vi "Chessy_Drive_Main.vi"(0 "Speed_Main":dbl, 1 "Turning_Main":dbl, 5 "Speed_Limit":dbl, 7 "Turning_Limit":dbl, 12 "Quick_Turn":bool) -> (3 "Left_Motor":dbl format="%.2f", 14 "Right_Motor":dbl format="%.2f")   [LabVIEW 2013]
panel:
  in  "Turning Scale":dbl=1.5
  in  "Turning Y":dbl[](array[numeric])=[-1.0, -0.5, -0.21, 0.0, 0.0, 0.0, 0.21, 0.5, 1.0]
  in  "Turning X":dbl[](array[numeric])=[-1.0, -0.75, -0.155, -0.15, 0.0, 0.15, 0.155, 0.75, 1.0]
  in  "Speed Y":dbl[](array[numeric])=[-1.0, -0.5, -0.21, 0.0, 0.0, 0.0, 0.21, 0.5, 1.0]
  in  "Speed X":dbl[](array[numeric])=[-1.0, -0.75, -0.155, -0.15, 0.0, 0.15, 0.155, 0.75, 1.0]
  in  "Turning_Hyd_Deadband":dbl=0.75
  in  "Speed_Hyd_Deadband":dbl=0.75
  out "Delta":dbl format="%.2f"
  # "Chessy Drive"
  # "This subystem takes turning and speed controls from a xbox joystick \nand creats left and right motor values"
  # "Tunning"
  # "Inputs"
  # "Test Points"
  # "Ouputs"
  # "Joystick Map (Lookup Table)"
  # "Hyp Cmd Deadband"
  # "Turning Power Mode"
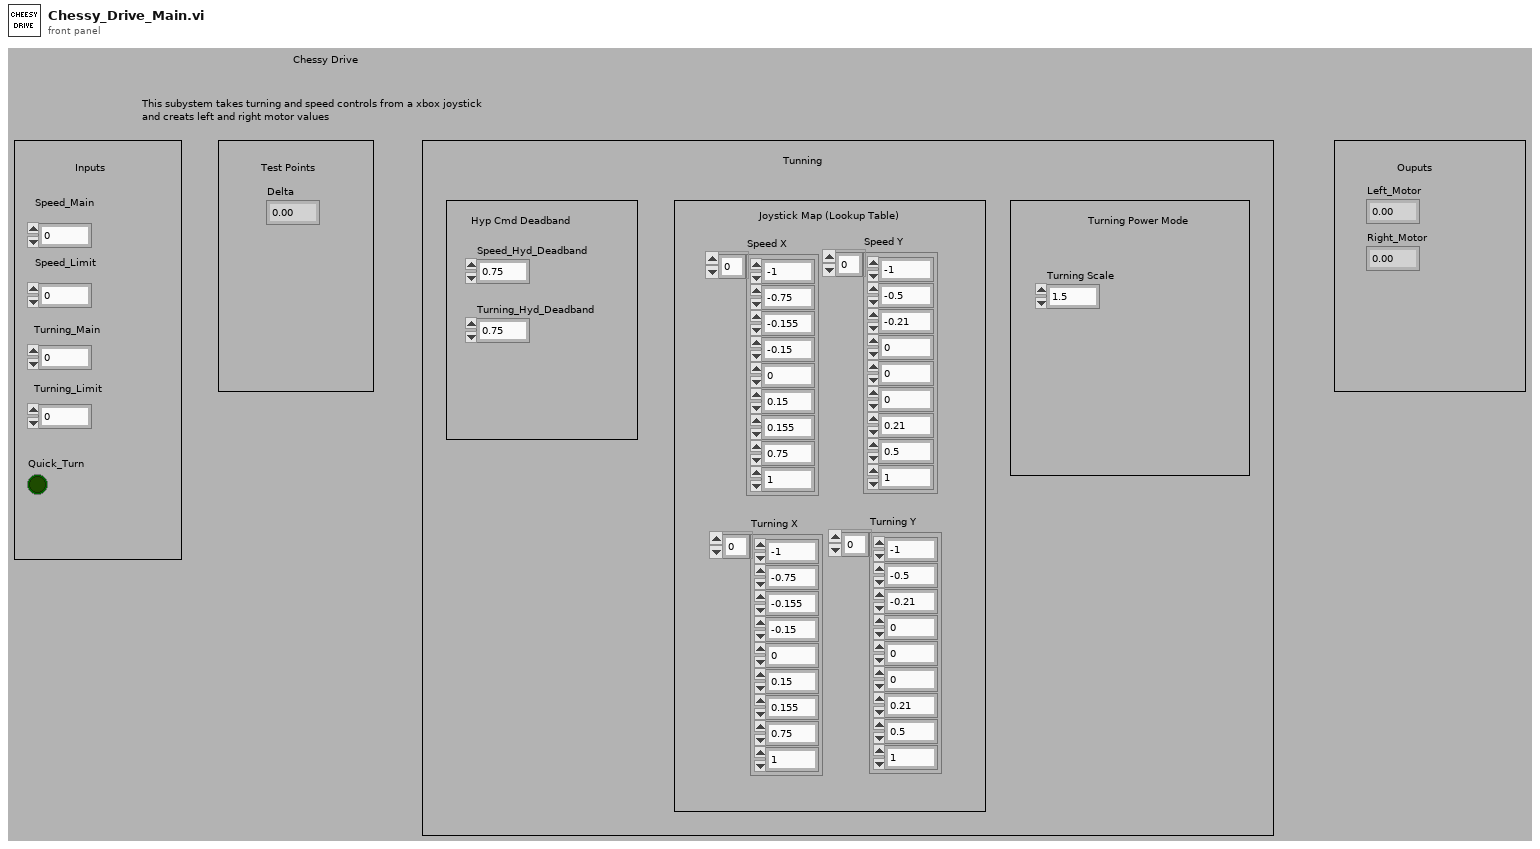
[diagram p1: front panel]
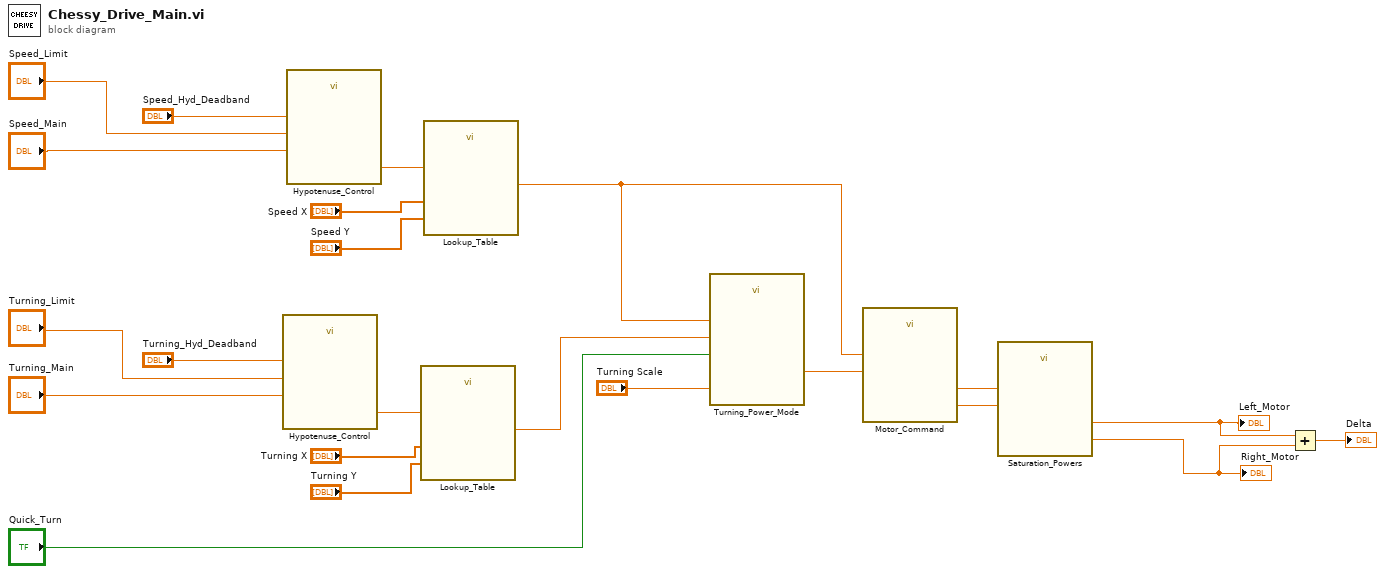
[diagram p0: block diagram]
diagram:
  n1 = call "Hypotenuse_Control.vi"("Deadband"="Turning_Hyd_Deadband", "Limit_Axis"="Turning_Limit", "Main_Axis"="Turning_Main") -> ("Axis_Adj"=w4:dbl)  [unwired: 8 in]
  n2 = call "Hypotenuse_Control.vi"("Deadband"="Speed_Hyd_Deadband", "Limit_Axis"="Speed_Limit", "Main_Axis"="Speed_Main") -> ("Axis_Adj"=w8:dbl)  [unwired: 8 in]
  n3 = call "Lookup_Table.vi"("Y_Array"="Turning Y", "x_in"=w4, "X_Array"="Turning X") -> ("y_out"=w14:dbl)  [unwired: 6 in]
  n4 = call "Lookup_Table.vi"("Y_Array"="Speed Y", "x_in"=w8, "X_Array"="Speed X") -> ("y_out"=w15:dbl)  [unwired: 6 in]
  n5 = call "Turning_Power_Mode.vi"("Turning_Scale"="Turning Scale", "Quick_Turn"="Quick_Turn", "Turning"=w14, "Power"=w15) -> ("Turning_Correction"=w18:dbl)  [unwired: 7 in]
  n6 = call "Motor_Command.vi"("Turning"=w18, "Power"=w15) -> ("Right_Motor"=w21:dbl, "Left_Motor"=w19:dbl)  [unwired: 8 in]
  n7 = call "Saturation_Powers.vi"("Right_Motor"=w21, "Left_Motor"=w19) -> ("Right_Motor_Say"=w16:dbl, "Left_Motor_Sat"=w17:dbl)  [unwired: 8 in]
  "Left_Motor" <- w17
  "Right_Motor" <- w16
  n8 = Add(x=w17, y=w16) -> (x+y=→"Delta":dbl)
